vi "visiontest.vi"() -> ()   [LabVIEW 2025]
uses:
  <vilib>/numeric/Random Number (Range) U64.vi
  <vilib>/numeric/sub_Random U32.vi
panel:
  out "Image Pixels (U16)":u16[][](array[numeric])
  out "error out 2":errorcluster
  in  "error in (no error)":errorcluster
  in  "Image Type":T1 items=["Grayscale (U8)", "Grayscale (I16)", "Grayscale (SGL)", "Complex (CSG)", "RGB (U32)", "HSL (U32)", "RGB (U64)", "Grayscale (U16)"]
  in  "Border Size":i32=3
  out "Array":u16[][](array[numeric])
  out "error out":errorcluster
  out "Image":T2(plugin-control)
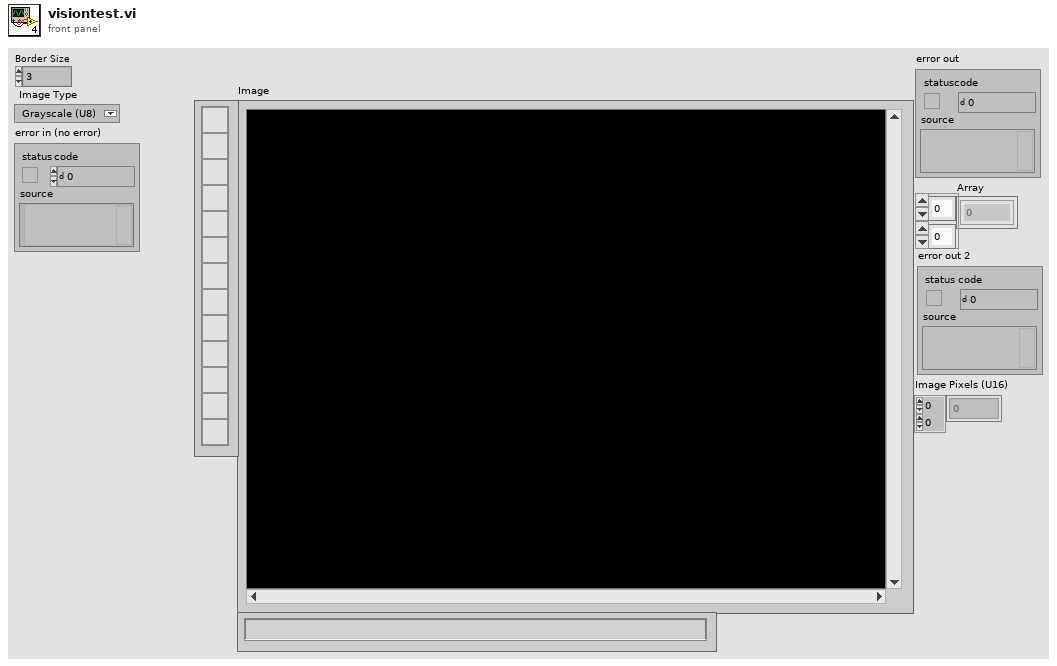
[diagram p1: front panel]
types:
  T1 = typedef "Image Type" = u32
  T2 = typedef "IMAQ Image.ctl" = refnum<image>
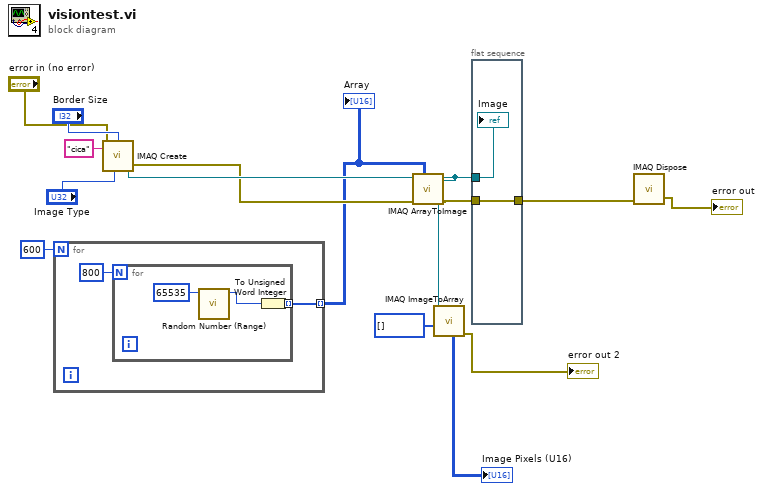
[diagram p0: block diagram]
diagram:
  n1 = for {
    N: 600 -> [_]
    tunnel: [w16] -> w8 mode=indexing
    n2 = for {
      N: 800 -> [_]
      tunnel: [w18] -> w16 mode=indexing
      n3 = call-poly <vilib>:"Random Number (Range).vi"("upper bound (100)"=u64 65535) -> ("number"=w19:u64)  [unwired: 10 in]
      n4 = To Unsigned Word Integer(number=w19) -> (unsigned 16bit integer=w18:u16)
    }
  }
  "Array" <- w8
  n5 = call "IMAQ Create"("Border Size"="Border Size", "Image Name"="cica", "Image Type"="Image Type", "error in (no error)"="error in (no error)") -> ("New Image"=w14:T2, "error out"=w10:errorcluster)  [unwired: 1 in]
  n6 = call "IMAQ ArrayToImage"("Image Pixels (U16)"=w8, "error in (no error)"=w10, "Image"=w14) -> ("error out"=w11:errorcluster, "Image Out"=w4:T2)  [unwired: 7 in]
  n7 = call "IMAQ ImageToArray"("Optional Rectangle"=i32[] [], "Image"=w4) -> ("Image Pixels (U16)"=→"Image Pixels (U16)":u16[][], "error out"=→"error out 2":errorcluster)  [unwired: 2 in, 3 out]
  n8 = flat-sequence {
    tunnel: w4 -> [w21]
    tunnel: [w22] -> w12
    tunnel: w11 -> [w22]
    frame #0 {
      "Image" <- w21
    }
  }
  n9 = call "IMAQ Dispose"("error in (no error)"=w12) -> ("error out"=→"error out":errorcluster)  [unwired: 5 in]
